vi "$CTL_Limit Check.vi"(8 "E-Stop":bool, 9 "Limit":dbl, 11 "X":dbl) -> (1 "X< Neg":bool, 2 "Neg <X<Pos":bool, 3 "X>Pos":bool)   [LabVIEW 2024]
doc: "X>Pos is TRUE if the X is greater than Pos Limit\nX<Pos is TRUE if the X is Less than Neg Limit\nNeg <X< Pos is TRUE when X is between the two limits"
panel:
  in  "Resets":i32
  out "Numeric":i32
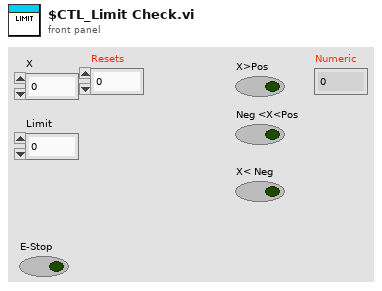
[diagram p1: front panel]
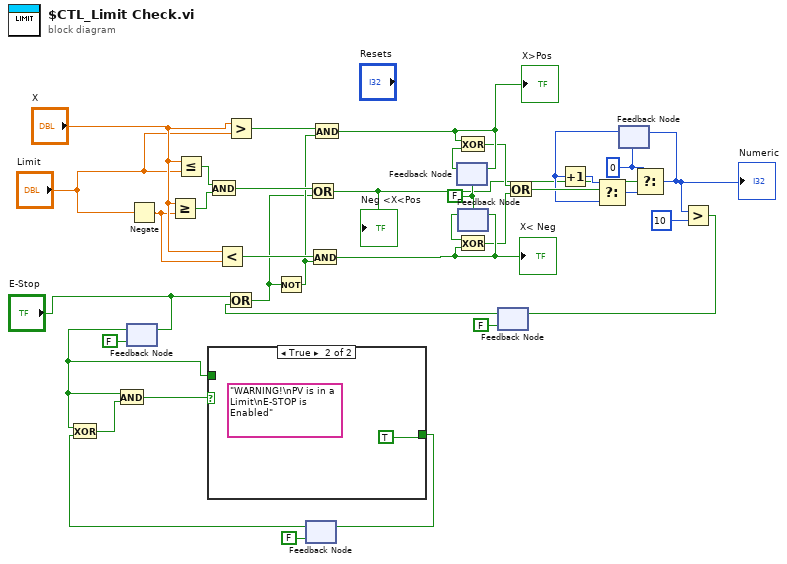
[diagram p0: block diagram]
diagram:
  w5 = FALSE ("x .or. y?")
  w12 = 0 ("t")
  n1 = feedback-in #1("E-Stop") -> ()
  n2 = feedback #1(FALSE ("E-Stop")) -> (w1:bool)
  n3 = Negate(x="Limit") -> (-x=w28:dbl)
  n4 = Greater Or Equal?(x="X", y=w28) -> (x >= y?=w35:bool)
  n5 = Less Or Equal?(x="X", y="Limit") -> (x <= y?=w36:bool)
  n6 = And(x=w36, y=w35) -> (x .and. y?=w32:bool)
  n7 = Less?(x="X", y=w28) -> (x < y?=w33:bool)
  n8 = Greater?(x="X", y="Limit") -> (0:w31:bool)
  n9 = feedback #2(FALSE) -> (w23:bool)
  n10 = Exclusive Or(1:w23, 2:w1) -> (0:w24:bool)
  n11 = And(x=w1, y=w24) -> (x .and. y?=w25:bool)
  n12 = case shown="True" w25 {
    tunnel: [w37 TRUE] -> w27
    tunnel: w1 -> [w37 _]
    frame False {
    }
    frame True {
      (unwired) "WARNING!\nPV is in a Limit\nE-STOP is Enabled" ("message")
    }
  }
  n13 = feedback-in #2(w27) -> ()
  n14 = feedback #3(w5) -> (w21:bool)
  n15 = feedback #4(w5) -> (w19:bool)
  n16 = feedback #5(FALSE) -> (w7:bool)
  n17 = Or(x="E-Stop", y=w7) -> (x .or. y?=w9:bool)
  n18 = Not(x=w9) -> (.not. x?=w30:bool)
  n19 = Or(x=w32, y=w9) -> (x .or. y?=w4:bool)
  "Neg <X<Pos" <- w4
  n20 = And(x=w33, y=w30) -> (x .and. y?=w20:bool)
  "X< Neg" <- w20
  n21 = And(x=w31, y=w30) -> (x .and. y?=w22:bool)
  "X>Pos" <- w22
  n22 = feedback-in #3(w22) -> ()
  n23 = Exclusive Or(1:w21, 2:w22) -> (0:w17:bool)
  n24 = feedback-in #4(w20) -> ()
  n25 = Exclusive Or(1:w20, 2:w19) -> (0:w18:bool)
  n26 = Or(x=w17, y=w18) -> (x .or. y?=w16:bool)
  n27 = feedback #6(w12) -> (w11:i32)
  n28 = Increment(x=w11) -> (x+1=w15:i32)
  n29 = Select(t=w15, s=w16, f=w11) -> (s? t:f=w14:i32)
  n30 = Select(t=w12, s=w4, f=w14) -> (s? t:f=w13:i32)
  "Numeric" <- w13
  n31 = feedback-in #6(w13) -> ()
  n32 = Greater?(x=w13, y=10) -> (0:w8:bool)
  n33 = feedback-in #5(w8) -> ()
